vi "Chamber controller Nov 21 2016.vi"() -> ()   [LabVIEW 2014]
uses:
  <vilib>/Instr/_visa.llb/VISA Configure Serial Port (Instr).vi
  Environmental Chamber LabVIEW and Instruments/Drivers and Software/Keithley 2100 Series/Public/Configure/Configure 2 Wire Resistance.vi
  <vilib>/Utility/file.llb/Write To Spreadsheet File (string).vi
  <vilib>/Utility/file.llb/Read From Spreadsheet File (string).vi
  Environmental Chamber LabVIEW and Instruments/Drivers and Software/keithley_6430/Keithley 6430/Public/Data/Read (Single Point).vi
  Environmental Chamber LabVIEW and Instruments/Drivers and Software/LabVIEW 8.2 Drivers/keithley_24xx/Keithley 24XX/Public/Data/Read (Single Point).vi
  Environmental Chamber LabVIEW and Instruments/Drivers and Software/keithley_24xx/Keithley 24XX/Keithley 24XX.lvlib
  Environmental Chamber LabVIEW and Instruments/Drivers and Software/keithley_6430/Keithley 6430/Keithley 6430.lvlib
  Environmental Chamber LabVIEW and Instruments/Drivers and Software/Keithley 2100 Series/Keithley 2100 Series.lvlib
panel:
  in  "Arduino COMs":T1={"Arduino 1"="COM23", "Arduino 2"="COM24", "Arduino 3"="COM25", "Arduino 4"="COM26", "Arduino 5"="COM27", "Arduino 6"="COM28"}
  out "saving data?":bool
  out "ArduinoQCM\ncluster":T2 caption="Arduino QCM" {"6" format="%#_10g"; "5" format="%#_10g"; "4" format="%#_10g"; "3" format="%#_10g"; "2" format="%#_10g"; "1" format="%#_10g"}
  in  "Data logging settings":T3={"Save during sequence only"=TRUE, "Save now"=FALSE, "sec between data points"=0.0, "Current data file path"=path "", "Save sample names"={"QCM1"="", "QCM2"="", "QCM3"="", "QCM4"="", "QCM5"="", "QCM6"="", "SRS"="", "K-2420"="", "K-6430"="", "K-2100"=""}, "Experiment Notes"=""} {"sec between data points" min=0.0 max=30.0 format="%#_13g"}
  in  "Sequence cluster":T4={"Save sequence"=FALSE, "Clear sequence"=FALSE, "Import sequence file"=FALSE, "Tare elapsed time"=TRUE, "Run Sequence"=FALSE, "Stop program when sequence ends"=TRUE, "User-defined\nsequence"=[], "Sequence end time"="", "Sequence\npreview"=[], "Current\nstep"=0, "Jump to next step"=FALSE} caption="Sequence settings"
  in  "Pressure parameters cluster":T5={"valve % open"=100.0, "Desired pressure"=0.0, "Vapor sccm"=0.0, "Gas sccm"=0.0, "Valve mode"=enum."% Open", "Pressure Mode"=enum."Abs. pressure", "analyte partial pressure"=23.8, "Turbo pump\nauto on"=TRUE, "Valve position (%)"=0.0, "read pressure"=0.0, "read vapor flow"=0.0, "read gas flow"=0.0, "pressure chart"={"pressure"=0.0}} caption="Pressure settings" {"read gas flow" format="%#_3g"; "read vapor flow" format="%#_3g"; "read pressure" format="%#_7f"; "Valve position (%)" format="%#_3g"; "analyte partial pressure" min=0.0 max=100.0 step=5.0; "Gas sccm" min=0 max=200 step=5; "Vapor sccm" min=0 max=200 step=5; "Desired pressure" min=0.0 max=760.0 step=5.0; "valve % open" min=0.0 max=100.0 step=5.0 format="%#_2f"}
  out "J-KEM temp chart":dbl(graph)
  out "Elapsed time (min)":dbl
  out "State date/time":string caption="Start time"
  out "K-2100 (Ohm)":cluster{"Measurement":dbl}(graph) caption="K-2100 Ohm"
  out "K-6430":cluster{"Measurement":dbl}(graph)
  out "K-2420":cluster{"Resistance":sgl}(graph)
  in  "Gate time (sec)":enum16{"0.1", "1.0 ", "10"}(ring)=enum."1.0 "
  out "MHz":dbl format="%.7f"
  out "QCM plot":T6(graph)
  in  "Stop":bool
  in  "Clear all charts":bool
  out "O2 sensor output":dbl[](array[numeric]) caption="atm\nTorr"
  in  "rapidox O2 Sensor":bool
  in  "setnag O2 Pump":bool
  in  "Baud Rate 2":i32(ring)=2 items=["2400", "4800", "9600", "19200", "38400", "57600", "115200"]
  in  "Com Port":i32(ring) items=["Com 1", "Com 2", "Com 3", "Com 4", "Com 5", "Com 6", "COM 7", "COM 8", "COM 9", "COM 10", "COM 11", "COM 12", "com 13", "COM 14"]
  in  "Com Port 2":i32(ring) items=["Com 1", "Com 2", "Com 3", "Com 4", "Com 5", "Com 6", "COM 7", "COM 8", "COM 9", "COM 10", "COM 11", "COM 12", "com 13", "COM 14"]
  out "Waveform Chart":cluster{dbl}(graph)
  out "O2 Concentration (PPM)":dbl
  out "Waveform Chart 6":cluster{dbl}(graph)
  # "Currently Unused"
  # "100%"
  # "SRS"
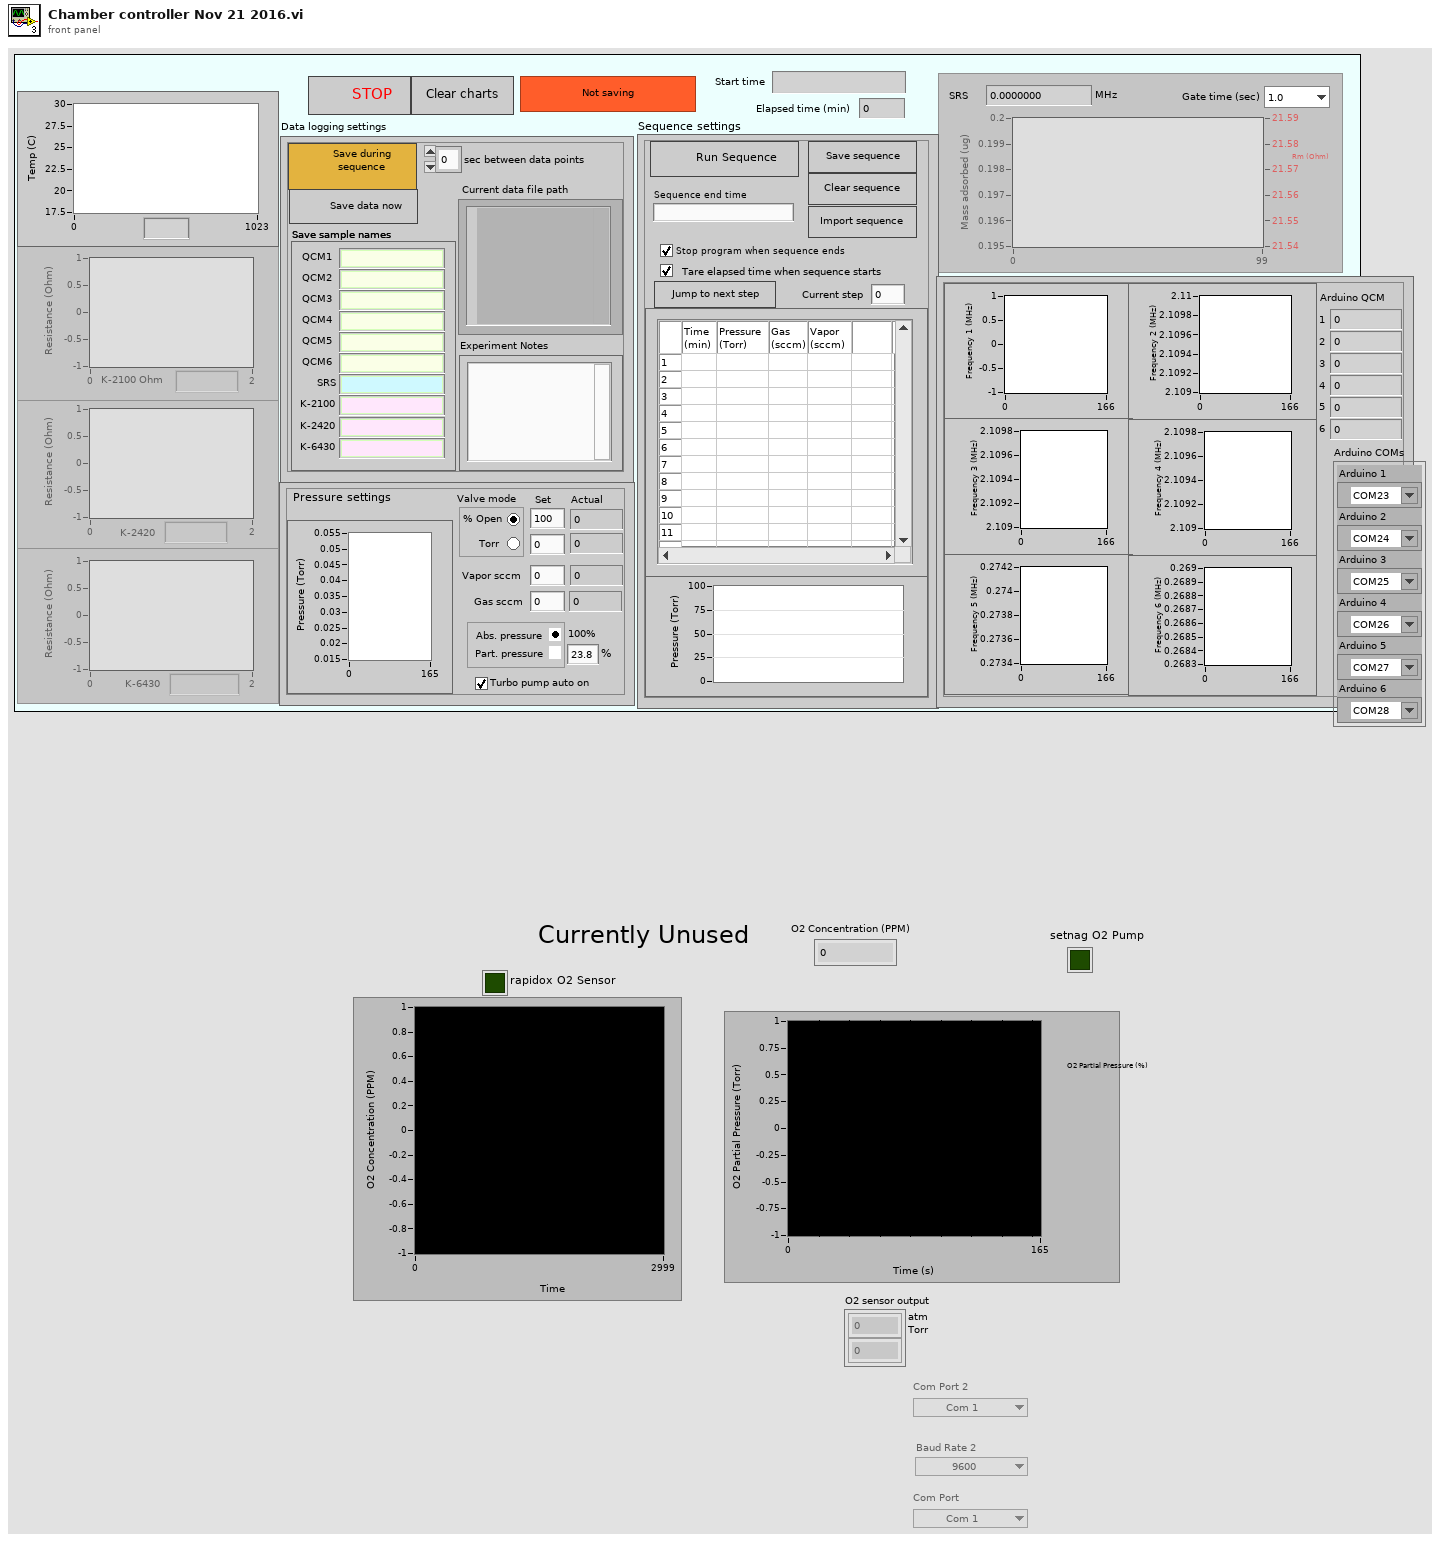
[diagram p1: front panel]
types:
  T1 = cluster{"Arduino 1":refnum<visa-resource-name>, "Arduino 2":refnum<visa-resource-name>, "Arduino 3":refnum<visa-resource-name>, "Arduino 4":refnum<visa-resource-name>, "Arduino 5":refnum<visa-resource-name>, "Arduino 6":refnum<visa-resource-name>}
  T2 = cluster{"arduino qcm 1":dbl, "1":dbl, "arduino qcm 2":dbl, "2":dbl, "arduino qcm 3":dbl, "3":dbl, "arduino qcm 4":dbl, "4":dbl, "arduino qcm 5":dbl, "5":dbl, "arduino qcm 6":dbl, "6":dbl}
  T3 = cluster{"Save during sequence only":bool, "Save now":bool, "sec between data points":dbl, "Current data file path":path, "Save sample names":cluster{"QCM1":string, "QCM2":string, "QCM3":string, "QCM4":string, "QCM5":string, "QCM6":string, "SRS":string, "K-2420":string, "K-6430":string, "K-2100":string}, "Experiment Notes":string}
  T4 = cluster{"Save sequence":bool, "Clear sequence":bool, "Import sequence file":bool, "Tare elapsed time":bool, "Run Sequence":bool, "Stop program when sequence ends":bool, "User-defined\nsequence":string[][], "Sequence end time":string, "Sequence\npreview":cluster{dbl[], dbl[]}[], "Current\nstep":i32, "Jump to next step":bool}
  T5 = cluster{"valve % open":dbl, "Desired pressure":dbl, "Vapor sccm":sgl, "Gas sccm":sgl, "Valve mode":enum32{"% Open", "Torr "}, "Pressure Mode":enum32{"Abs. pressure", " Part. pressure"}, "analyte partial pressure":dbl, "Turbo pump\nauto on":bool, "Valve position (%)":dbl, "read pressure":dbl, "read vapor flow":dbl, "read gas flow":dbl, "pressure chart":cluster{"pressure":dbl}}
  T6 = cluster{"Numeric Control":dbl, "Resistance out":dbl}
  T7 = cluster{"Keithley 6430":bool, "J-KEM":bool, "Keithley 2420":bool, "Keithley 2100":bool, "SRS QCM":bool, "Pressure control":bool, "Arduino":bool}
  T8 = enum8{"Enabled", "Disabled", "Disabled and Grayed Out"}
  T9 = enum16{"open", "open or create", "create or replace", "create", "open (read only)"}
  T10 = enum16{"no parity", "odd parity", "even parity", "mark parity", "space parity"}
  T11 = cluster{"f":dbl, "f":dbl, "f":dbl, "f":dbl, "f":dbl, "f 2":dbl}
  T12 = cluster{"String":string, "String":string, "String":string}
  T13 = cluster{"task out":refnum<k21>, "error out":errorcluster, "task out":refnum<k21>, "error out":errorcluster, "task out":refnum<k21>, "error out":errorcluster, "VISA resource name":refnum<visa-resource-name>, "error out":errorcluster}
  T14 = cluster{"task out":refnum<k21>, "error out":errorcluster, "task out":refnum<k21>, "error out":errorcluster, "task out":refnum<k21>, "error out":errorcluster, "VISA resource name out":refnum<visa-resource-name>, "error out":errorcluster}
  T15 = cluster{bool, "VISA resource name":refnum<visa-resource-name>, "error out":errorcluster}
  T16 = cluster{bool, "VISA resource name out":refnum<visa-resource-name>, "error out":errorcluster}
  T17 = cluster{"VISA resource name out":refnum<visa-resource-name>, "error out":errorcluster, "VISA resource name out":refnum<visa-resource-name>, "error out":errorcluster, "VISA resource name out":refnum<visa-resource-name>, "error out":errorcluster, "VISA resource name out":refnum<visa-resource-name>, "error out":errorcluster, "VISA resource name out":refnum<visa-resource-name>, "error out":errorcluster, "VISA resource name out 2":refnum<visa-resource-name>, "error out 2":errorcluster}
  T18 = cluster{bool, cluster{"task out":refnum<k21>, "error out":errorcluster, "task out":refnum<k21>, "error out":errorcluster, "task out":refnum<k21>, "error out":errorcluster, "VISA resource name out":refnum<visa-resource-name>, "error out":errorcluster}}
  T19 = cluster{"Boolean":bool, "VISA resource name out":refnum<visa-resource-name>, "error out":errorcluster}
  T20 = cluster{bool, "VISA out":refnum<visa-resource-name>, "error out":errorcluster}
  T21 = cluster{"Boolean":bool, "VISA out":refnum<visa-resource-name>, "error out":errorcluster}
  T22 = cluster{"Numeric Control":dbl, "Cluster":cluster{"Numeric Control":dbl}, "String":string, "error out":errorcluster}
  T23 = cluster{bool, "Com Port":i32, "Numeric Control out":dbl}
  T24 = cluster{"Arduino address":refnum<visa-resource-name>, "error in (no error)":errorcluster, "Arduino address 2":refnum<visa-resource-name>, "error in (no error) 2":errorcluster, "Arduino address 3":refnum<visa-resource-name>, "error in (no error) 3":errorcluster, "Arduino address 4":refnum<visa-resource-name>, "error in (no error) 4":errorcluster, "Arduino address 5":refnum<visa-resource-name>, "error in (no error) 5":errorcluster, "Arduino address 6":refnum<visa-resource-name>, "error in (no error) 6":errorcluster}
  T25 = cluster{"mean":string, "mean":string, "mean":string, "mean":string, "mean":string, "mean":string}
  T26 = cluster{"String data out":string, string, string, string}
  T27 = cluster{"valve % open":dbl, "Desired pressure":dbl, "Vapor sccm":sgl, "Gas sccm":sgl, "Valve mode":enum32{"% Open", "Torr "}, "Pressure Mode":enum32{"Abs. pressure", " Part. pressure"}, "analyte partial pressure":dbl, "Turbo pump\nauto on":bool}
  T28 = cluster{"User-defined\nsequence":string[][], "Present (s)":dbl, "current  step # in":i32, "sequence end time in":timestamp}
  T29 = cluster{"current  step # in":i32, "sequence end time in":timestamp, "Boolean":bool}
  T30 = cluster{"press/RH/gas/vapor":cluster{"pressure":string, "RH":string, "gas flow":string, "vapor flow":string}, "Cluster":cluster{"Valve position (%)":dbl, "read pressure":dbl, "read vapor flow":dbl, "read gas flow":dbl}}
  T31 = cluster{"Boolean":bool, "DAQ IDs in":cluster{"task out":refnum<k21>, "error out":errorcluster, "task out":refnum<k21>, "error out":errorcluster, "task out":refnum<k21>, "error out":errorcluster, "VISA Refnum out":refnum<visa-resource-name>, "error out":errorcluster}}
  T32 = cluster{"mean":dbl, "mean":dbl, "mean":dbl, "mean":dbl, "mean":dbl, "mean":dbl}
  T33 = cluster{"f":dbl, "f":dbl, "f":dbl, "f":dbl, "f":dbl}[]
  T34 = cluster{"pressure":string, "RH":string, "gas flow":string, "vapor flow":string}
  T35 = cluster{"Valve position (%)":dbl, "read pressure":dbl, "read vapor flow":dbl, "read gas flow":dbl}
  T36 = cluster{dbl, dbl, dbl, dbl, dbl, dbl, dbl, dbl, dbl, dbl, dbl, dbl}
  T37 = cluster{"QCM1":string, "QCM2":string, "QCM3":string, "QCM4":string, "QCM5":string, "QCM6":string, "SRS":string, "K-2420":string, "K-6430":string, "K-2100":string}
  T38 = cluster{"task out":refnum<k21>, "error out":errorcluster, "task out":refnum<k21>, "error out":errorcluster, "task out":refnum<k21>, "error out":errorcluster, "VISA Refnum out":refnum<visa-resource-name>, "error out":errorcluster}
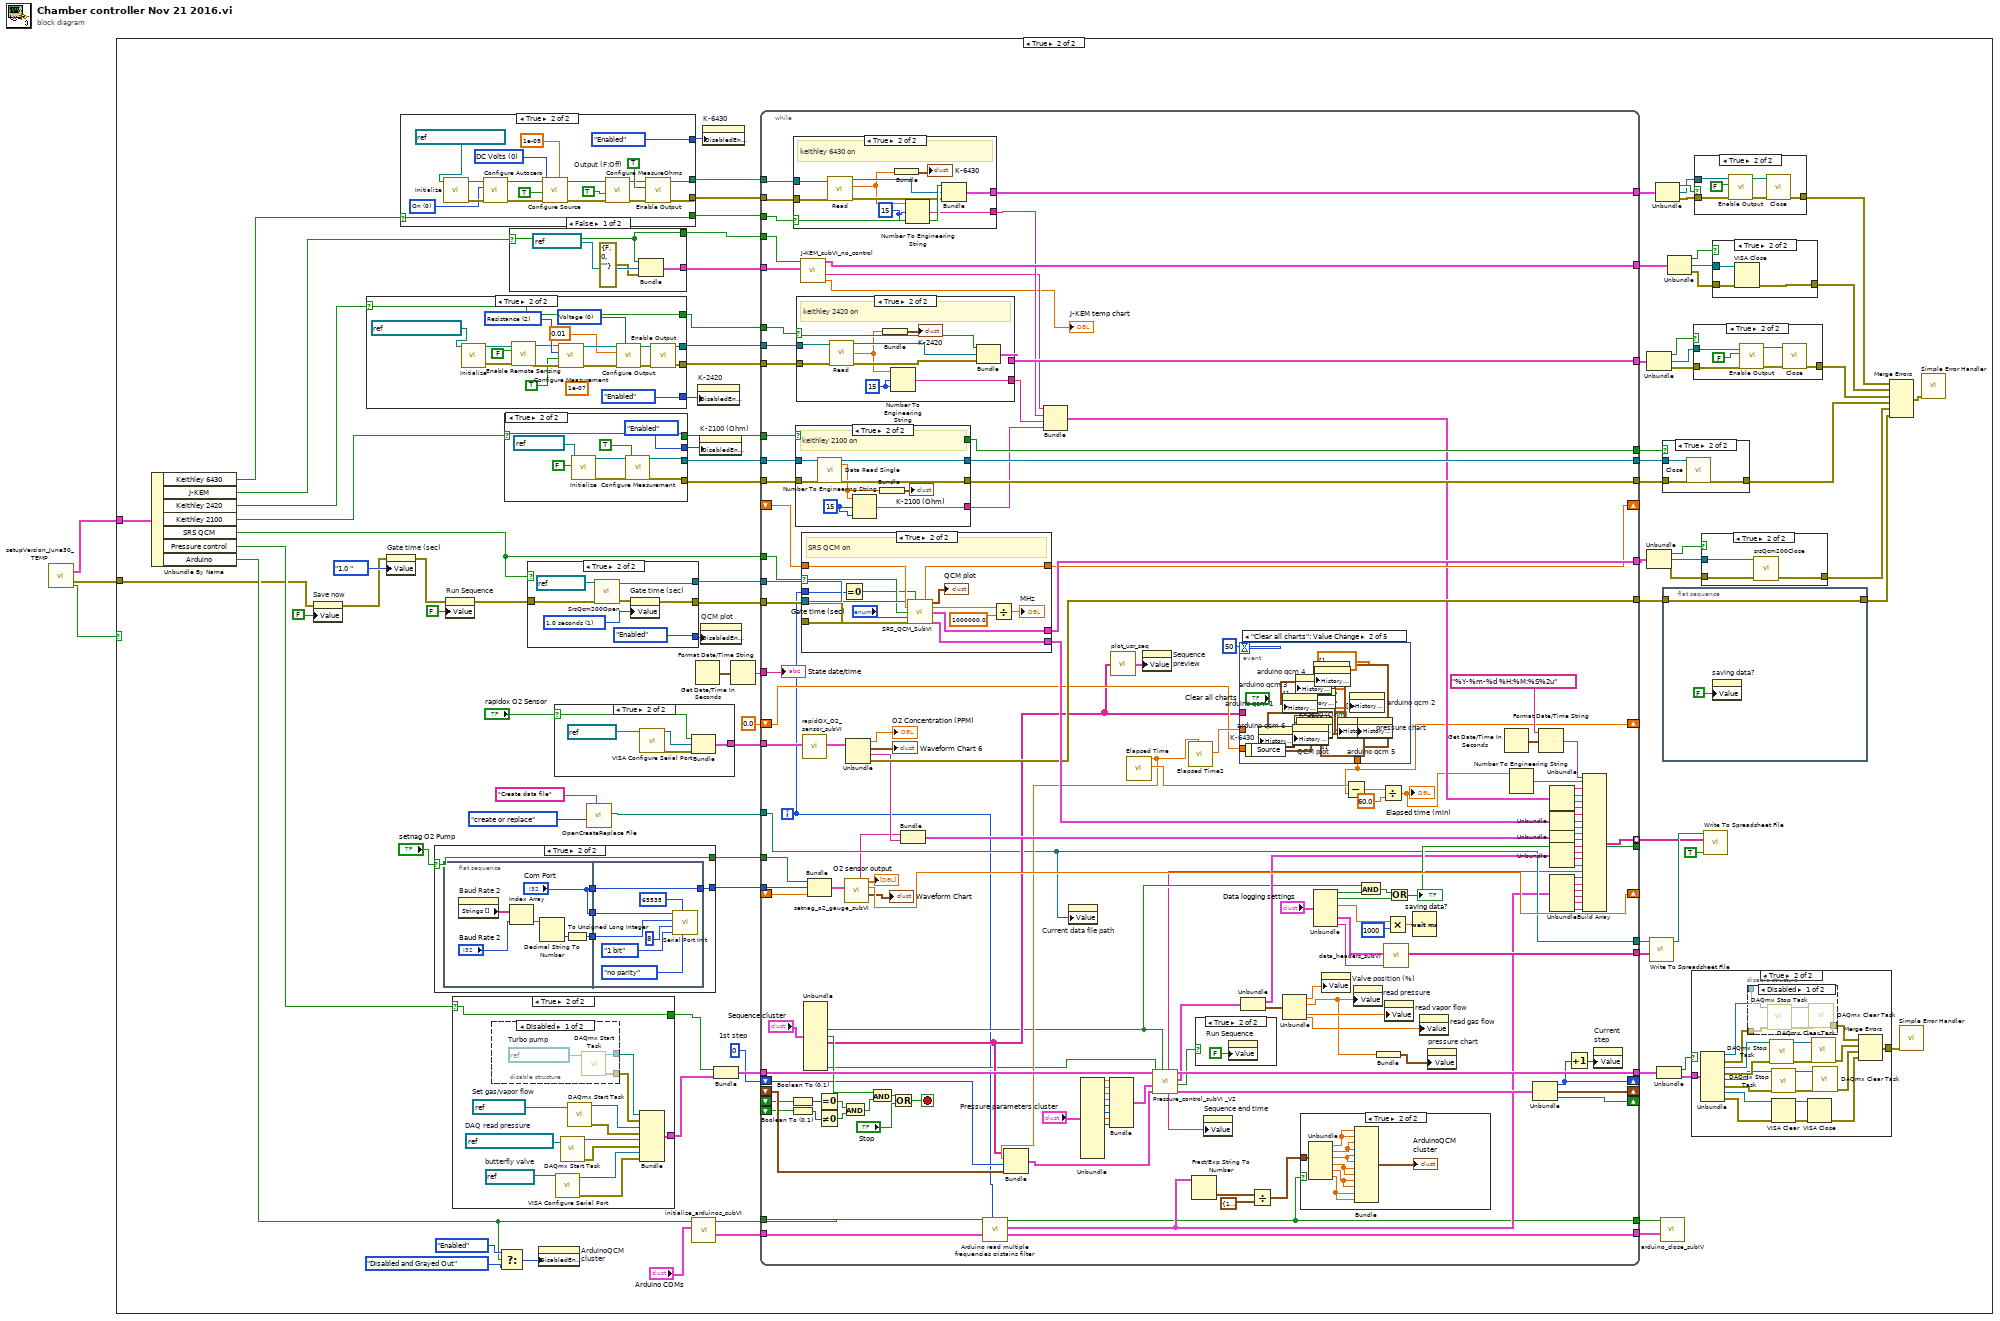
[diagram p0: block diagram]
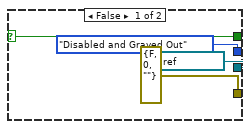
[diagram p4: hidden frame]
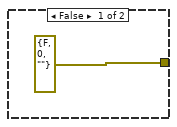
[diagram p5: hidden frame]
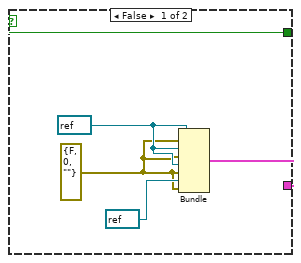
[diagram p7: hidden frame]
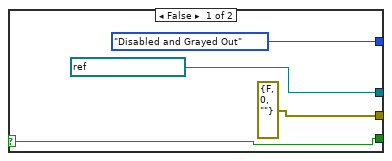
[diagram p10: hidden frame]
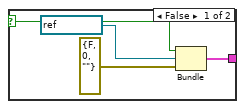
[diagram p11: hidden frame]
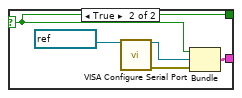
[diagram p13: hidden frame]
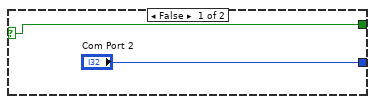
[diagram p14: hidden frame]
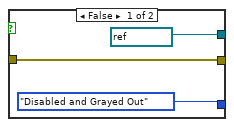
[diagram p16: hidden frame]
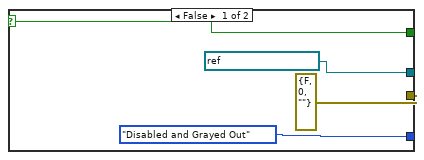
[diagram p18: hidden frame]
diagram:
  n1 = call "setupVersion_June30_TEMP.vi"() -> ("Instruments on/off"=w1:T7, "error IO"=w2:errorcluster, "OK"=w3:bool)  [unwired: 13 in]
  n2 = case shown="True" w3 {
    tunnel: w2 -> [_ w8]
    tunnel: w1 -> [_ w16]
    frame False {
    }
    frame True {
      w28 = 0  # 1st step
      n3 = Unbundle By Name(w16) -> ("Keithley 6430"=w15:bool, "J-KEM"=w14:bool, "Keithley 2420"=w13:bool, "Keithley 2100"=w12:bool, "SRS QCM"=w11:bool, "Pressure control"=w10:bool, "Arduino"=w9:bool)
      n4 = property on="Save now" class="Bool (strict)"(error in=w8, "Value"=FALSE) -> (error out=w7:errorcluster)  [unwired: 1 in, 1 out]
      n5 = case shown="True" w13 {
        selector: w13 -> [w254 w258]
        tunnel: [refnum<visa-resource-name> "GPIB1::24::INSTR" ("VISA resource name") w267] -> w92
        tunnel: [errorcluster {"status"=FALSE, "code"=0, "source"=""} ("error out") w262] -> w91
        tunnel: [T8."Disabled and Grayed Out" ("Disabled") T8."Enabled" ("Disabled")] -> w55
        tunnel: [w254 w258] -> w48
        frame False {
        }
        frame True {
          (unwired) 1e-07 ("Manual Range (1.0)")
          w269 = u16 0 items=["Voltage", "Current"] ("Source Mode  (0: Voltage)")
          w274 = u16 2 items=["Volts", "Current", "Resistance"] ("Function (0: Volts)")
          n6 = call "Initialize.vi"("VISA resource name"=refnum<visa-resource-name> "GPIB1::24::INSTR") -> ("error out"=w263:errorcluster, "VISA resource name out"=w266:refnum<visa-resource-name>)  [unwired: 9 in]
          n7 = call "Enable Remote Sensing.vi"("error in (no error)"=w263, "Enable Remote Sensing (T: Enable)"=FALSE ("4-wire?"), "VISA resource name"=w266) -> ("error out"=w264:errorcluster, "VISA resource name out"=w265:refnum<visa-resource-name>)  [unwired: 7 in]
          n8 = call "Configure Measurement.vi"("error in (no error)"=w264, "Enable Auto Range (T:Enable)"=TRUE, "Function (0: Volts)"=w274, "VISA resource name"=w265) -> ("error out"=w273:errorcluster, "VISA resource name out"=w272:refnum<visa-resource-name>)  [unwired: 6 in]
          n9 = call "Configure Output.vi"("Source Mode  (0: Voltage)"=w269, "error in (no error)"=w273, "Output Level (0)"=0.01 ("Applied Voltage (V)"), "VISA resource name"=w272) -> ("error out"=w271:errorcluster, "VISA resource name out"=w270:refnum<visa-resource-name>)  [unwired: 6 in]
          n10 = call "Enable Output.vi"("error in (no error)"=w271, "VISA resource name"=w270) -> ("error out"=w262:errorcluster, "VISA resource name out"=w267:refnum<visa-resource-name>)  [unwired: 8 in]
        }
      }
      n11 = property on="Gate time (sec)" class="Enum (strict)"(error in=w7, "Value"=enum16{"0.1", "1.0 ", "10"}."1.0 " ("Gate time (sec)")) -> (error out=w17:errorcluster)  [unwired: 1 in, 1 out]
      n12 = case shown="True" w15 {
        selector: w15 -> [w168 w172]
        tunnel: [refnum<visa-resource-name> "GPIB0::29::INSTR" ("VISA resource name") w185] -> w61
        tunnel: [errorcluster {"status"=FALSE, "code"=0, "source"=""} ("error out") w186] -> w60
        tunnel: [T8."Disabled and Grayed Out" ("Disabled") T8."Enabled" ("Disabled")] -> w54
        tunnel: [w168 w172] -> w47
        frame False {
        }
        frame True {
          w174 = u16 0 items=["DC Volts", "DC Current"] ("Source Function (0: DC Volts)")
          w181 = u16 0 items=["On", "Off", "Once"] ("Autozero  (0: On)")
          w189 = TRUE  # Output (F:Off)
          n13 = call "Initialize.vi"("VISA resource name"=refnum<visa-resource-name> "GPIB0::30::INSTR") -> ("error out"=w182:errorcluster, "VISA resource name out"=w183:refnum<visa-resource-name>)  [unwired: 4 in, 5 out]
          n14 = call "Configure Autozero.vi"("error in (no error)"=w182, "Autozero  (0: On)"=w181, "VISA resource name"=w183) -> ("error out"=w177:errorcluster, "VISA resource name out"=w179:refnum<visa-resource-name>)  [unwired: 7 in]
          n15 = call "Configure Source.vi"("I-Source Level [A]"=1e-09, "error in (no error)"=w177, "Auto Range (T:Enable)"=TRUE, "Source Function (0: DC Volts)"=w174, "VISA resource name"=w179) -> ("error out"=w176:errorcluster, "VISA resource name out"=w178:refnum<visa-resource-name>)  [unwired: 5 in]
          n16 = call "Configure MeasureOhms.vi"("error in (no error)"=w176, "Auto Range (T:Enable)"=TRUE, "VISA resource name"=w178) -> ("error out"=w190:errorcluster, "VISA resource name out"=w188:refnum<visa-resource-name>)  [unwired: 3 in, 4 out]
          n17 = call "Enable Output.vi"("error in (no error)"=w190, "Enable Output (F:Off)"=w189, "VISA resource name"=w188) -> ("error out"=w186:errorcluster, "VISA resource name out"=w185:refnum<visa-resource-name>)  [unwired: 7 out]
        }
      }
      n18 = case shown="True" "setnag O2 Pump" {
        selector: "setnag O2 Pump" -> [w213 w215]
        tunnel: ["Com Port 2" w216] -> w88
        tunnel: [w213 w215] -> w36
        frame False {
        }
        frame True {
          n19 = flat-sequence {
            tunnel: ["Com Port"] -> w219
            tunnel: [w221] -> w218
            tunnel: ["Com Port"] -> w217
            tunnel: w219 -> [w227]
            tunnel: w218 -> [w226]
            tunnel: w217 -> [w228]
            tunnel: [w228] -> w216
            frame #0 {
              n20 = property on="Baud Rate 2" class="Ring (strict)"() -> ("Strings []"=w223:string[])  [unwired: 2 in, 2 out]
              n21 = Index Array(array=w223, index="Baud Rate 2") -> (element=w224:string)
              n22 = Decimal String To Number(string=w224) -> (number=w222:i32)  [unwired: 2 in, 1 out]
              n23 = To Unsigned Long Integer(number=w222) -> (unsigned 32bit integer=w221:u32)
            }
            frame #1 {
              n24 = call <vilib>:"Serial Port Init.vi"("parity"=T10."no parity", "buffer size"=u16 65535, "stop bits"=enum16{"1 bit", "1.5 bits", "2 bits"}."1 bit", "data bits"=u16 8, "baud rate"=w226, "port number"=w227) -> ()  [unwired: 1 in, 1 out]
            }
          }
        }
      }
      n25 = property on="Run Sequence" class="Bool (strict)"(error in=w17, "Value"=FALSE) -> (error out=w23:errorcluster)  [unwired: 1 in, 1 out]
      n26 = case shown="True" w10 {
        selector: w10 -> [w140 w145]
        tunnel: [w141 w147] -> w30
        tunnel: [w140 w145] -> w31
        frame False {
          w143 = refnum<k21> refnum ("task out")
          w142 = errorcluster {"status"=FALSE, "code"=0, "source"=""} ("error out")
          n27 = Bundle("task out"=w143, "error out"=w142, "task out"=w143, "error out"=w142, "task out"=w143, "error out"=w142, "VISA resource name"=refnum<visa-resource-name> refnum, "error out"=w142) -> (w141:T13)  [unwired: 1 in]
        }
        frame True {
          w155 = refnum<visa-resource-name> "COM5"  # butterfly valve
          w156 = refnum<k21> "Setflow"  # Set gas/vapor flow
          w157 = refnum<k21> "AllDaqReadings"  # DAQ read pressure
          n28 = disable-structure shown="Disabled" {
            disable-tunnel: [w159 _] -> w154
            disable-tunnel: [w158 _] -> w153
            frame Disabled {
              w160 = refnum<k21> "TurboON"  # Turbo pump
              n29 = call <vilib>:"DAQmx Start Task.vi"("task/channels in"=w160) -> ("task out"=w159:refnum<k21>, "error out"=w158:errorcluster)  [unwired: 13 in]
            }
            frame Enabled {
            }
          }
          n30 = call-poly "VISA Configure Serial Port"("VISA resource name"=w155) -> ("VISA resource name out"=w148:refnum<visa-resource-name>, "error out"=w146:errorcluster)  [unwired: 13 in]
          n31 = call <vilib>:"DAQmx Start Task.vi"("task/channels in"=w157) -> ("task out"=w150:refnum<k21>, "error out"=w149:errorcluster)  [unwired: 13 in]
          n32 = call <vilib>:"DAQmx Start Task.vi"("task/channels in"=w156) -> ("task out"=w152:refnum<k21>, "error out"=w151:errorcluster)  [unwired: 13 in]
          n33 = Bundle("task out"=w154, "error out"=w153, "task out"=w152, "error out"=w151, "task out"=w150, "error out"=w149, "VISA resource name out"=w148, "error out"=w146) -> (w147:T14)  [unwired: 1 in]
        }
      }
      n34 = Select(t=T8."Enabled" ("Disabled"), s=w9, f=T8."Disabled and Grayed Out" ("Disabled")) -> (s? t:f=w22:T8)
      n35 = case shown="True" w12 {
        selector: w12 -> [w102 w107]
        tunnel: [refnum<visa-resource-name> "K-2100" ("VISA resource name out") w110] -> w45
        tunnel: [errorcluster {"status"=FALSE, "code"=0, "source"=""} ("error out") w109] -> w44
        tunnel: [w102 w107] -> w43
        tunnel: [T8."Disabled and Grayed Out" ("Disabled") T8."Enabled" ("Disabled")] -> w38
        frame False {
        }
        frame True {
          n36 = call "Initialize.vi"("VISA resource name"=refnum<visa-resource-name> "K-2100", "Reset? (T: Reset)"=FALSE) -> ("VISA resource name out"=w111:refnum<visa-resource-name>, "error out"=w108:errorcluster)  [unwired: 16 in]
          n37 = call-poly "Configure Measurement.vi"("VISA resource name"=w111, "error in (no error)"=w108, "Auto Range? (T: Auto)"=TRUE) -> ("VISA resource name out"=w110:refnum<visa-resource-name>, "error out"=w109:errorcluster)  [unwired: 15 in]
        }
      }
      n38 = case shown="False" w14 {
        selector: w14 -> [w204 w209]
        tunnel: [w205 w210] -> w77
        tunnel: [w204 w209] -> w71
        frame False {
          n39 = Bundle(w204, "VISA resource name"=refnum<visa-resource-name> "COM3", "error out"=errorcluster {"status"=FALSE, "code"=0, "source"=""}) -> (w205:T15)  [unwired: 1 in]
        }
        frame True {
          n40 = call-poly "VISA Configure Serial Port"("VISA resource name"=refnum<visa-resource-name> "COM3") -> ("VISA resource name out"=w211:refnum<visa-resource-name>, "error out"=w208:errorcluster)  [unwired: 13 in]
          n41 = Bundle(w209, "VISA resource name out"=w211, "error out"=w208) -> (w210:T16)  [unwired: 1 in]
        }
      }
      n42 = case shown="True" w11 {
        tunnel: [refnum<visa-resource-name> "COM6" ("VISA in") w243] -> w90
        tunnel: [w238 w240] -> w89
        tunnel: w23 -> [w238 w245]
        tunnel: [T8."Disabled and Grayed Out" ("Disabled") T8."Enabled" ("Disabled")] -> w56
        frame False {
        }
        frame True {
          w242 = u16 1 items=["0.1 seconds", "1.0 seconds", "10.0 seconds"] ("Gate time")
          n43 = call "SrsQcm200Open.vi"("error in"=w245, "VISA in"=refnum<visa-resource-name> "COM6") -> ("error out"=w241:errorcluster, "VISA out"=w243:refnum<visa-resource-name>)  [unwired: 3 in]
          n44 = property on="Gate time (sec)" class="Enum (strict)"(error in=w241, "Value"=w242) -> (error out=w240:errorcluster)  [unwired: 1 in, 1 out]
        }
      }
      n45 = property on="ArduinoQCM\ncluster" class="Clust (strict)"("DisabledEnum"=w22) -> ()  [unwired: 2 in, 2 out]
      n46 = case shown="True" "rapidox O2 Sensor" {
        selector: "rapidox O2 Sensor" -> [w191 w196]
        tunnel: [w192 w197] -> w67
        frame False {
          n47 = Bundle(w191, "VISA resource name"=refnum<visa-resource-name> "COM7", "error out"=errorcluster {"status"=FALSE, "code"=0, "source"=""}) -> (w192:T15)  [unwired: 1 in]
        }
        frame True {
          n48 = call-poly "VISA Configure Serial Port"("VISA resource name"=refnum<visa-resource-name> "COM7") -> ("VISA resource name out"=w198:refnum<visa-resource-name>, "error out"=w195:errorcluster)  [unwired: 13 in]
          n49 = Bundle(w196, "VISA resource name out"=w198, "error out"=w195) -> (w197:T16)  [unwired: 1 in]
        }
      }
      n50 = call "OpenCreateReplace File.vi"("prompt"="Create data file", "function (open:0)"=T9."create or replace") -> ("new file path"=w46:path)  [unwired: 6 in, 3 out]
      n51 = call "initialize_arduinos_subVI.vi"("arduino 1-6 addresses"="Arduino COMs", "arduinos on?"=w9) -> ("arduino addresses/errors"=w32:T17, "arduinos on/off"=w52:bool)  [unwired: 8 in]
      n52 = Get Date/Time In Seconds() -> (seconds since 1Jan1904=w94:timestamp)
      n53 = property on="K-2420" class="WFChart (strict)"("DisabledEnum"=w55) -> ()  [unwired: 2 in, 2 out]
      n54 = property on="K-2100 (Ohm)" class="WFChart (strict)"("DisabledEnum"=w38) -> ()  [unwired: 2 in, 2 out]
      n55 = property on="QCM plot" class="WFChart (strict)"("DisabledEnum"=w56) -> ()  [unwired: 2 in, 2 out]
      n56 = property on="K-6430" class="WFChart (strict)"("DisabledEnum"=w54) -> ()  [unwired: 2 in, 2 out]
      n57 = Bundle(w31, w30) -> (w29:T18)  [unwired: 1 in]
      n58 = Format Date/Time String(seconds (now)=w94) -> (date/time string=w35:string)  [unwired: 2 in]
      n59 = while {
        shift-right: [w421] -> _
        shift-left: _ -> [w349]
        tunnel: [w405] -> w53 mode=indexing if=w372
        tunnel: w48 -> [w410]
        tunnel: w92 -> [w420]
        tunnel: w91 -> [w419]
        tunnel: w90 -> [w418]
        tunnel: w89 -> [w417]
        tunnel: w11 -> [w416]
        tunnel: w36 -> [w351]
        tunnel: w88 -> [w352]
        tunnel: [w415] -> w85
        tunnel: [w414] -> w81
        tunnel: w77 -> [w413]
        tunnel: [w412] -> w76
        tunnel: w71 -> [w411]
        tunnel: w67 -> [w360]
        tunnel: [w356] -> w5
        tunnel: [w291] -> w66
        tunnel: w46 -> [w291]
        shift-right: [w403] -> _
        shift-left: _ -> [w404]
        tunnel: w61 -> [w409]
        tunnel: w60 -> [w408]
        tunnel: [w407] -> w59
        tunnel: [w372] -> _
        tunnel: w52 -> [w278]
        tunnel: w32 -> [w281]
        tunnel: [w277] -> w50
        tunnel: [w279] -> w51
        tunnel: [w391] -> w49
        tunnel: w47 -> [w384]
        tunnel: w45 -> [w371]
        tunnel: w44 -> [w370]
        tunnel: w43 -> [w369]
        tunnel: [w368] -> w42
        tunnel: [w367] -> w41
        tunnel: [w366] -> w40
        shift-right: [w343] -> _
        shift-left: 0.0 ("Elapsed Time (s)") -> [w344]
        tunnel: w35 -> [w334]
        tunnel: w29 -> [w316]
        shift-right: [w286] -> _
        shift-left: w28 -> [w305]
        shift-right: [w311] -> _
        shift-left: _ -> [w309]
        shift-right: [w310] -> _
        shift-left: _ -> [w308]
        shift-left: _ -> [w307]
        tunnel: [w303] -> w27
        i -> [w276]
        stop <- w374 stop-if-true
        n60 = Boolean To (0,1)(Boolean=w308) -> (0, 1=w382:i16)
        n61 = Boolean To (0,1)(Boolean=w307) -> (0, 1=w381:i16)
        n62 = case "Keithley 6430" shown="True" w384 {
          selector: w384 -> [w456 w467]
          tunnel: w409 -> [w455 w464]
          tunnel: w408 -> [w454 w463]
          tunnel: ["" w466] -> w355
          tunnel: [w453 w465] -> w407
          frame False {
            # "keithley 6430 off"
            n63 = Bundle(w456, "VISA resource name out"=w455, "error out"=w454) -> (w453:T16)  [unwired: 1 in]
          }
          frame True {
            w458 = i16 15 ("width (-)")
            # "keithley 6430 on"
            n64 = call-poly "Read.vi"("error in (no error)"=w463, "VISA resource name"=w464) -> ("error out"=w462:errorcluster, "Measurement"=w460:dbl, "VISA resource name out"=w461:refnum<visa-resource-name>)  [unwired: 1 in, 6 out]
            n65 = Bundle("Measurement"=w460) -> (→"K-6430":cluster{"Measurement":dbl})  [unwired: 1 in]
            n66 = Number To Engineering String(2:w458, 3:w458, 4:w460) -> (0:w466:string)  [unwired: 1 in]
            n67 = Bundle(w467, "VISA resource name out"=w461, "error out"=w462) -> (w465:T16)  [unwired: 1 in]
          }
        }
        n68 = case shown="True" w369 {
          selector: w369 -> [w432 w437]
          tunnel: [w433 w444] -> w367
          tunnel: [w434 w443] -> w366
          tunnel: w371 -> [w433 w442]
          tunnel: w370 -> [w434 w441]
          tunnel: ["" w439] -> w353
          tunnel: [w432 w437] -> w368
          frame False {
            # "keithley 2100 off"
          }
          frame True {
            w436 = i16 15 ("width (-)")
            # "keithley 2100 on"
            n69 = call "Data Read Single.vi"("VISA resource name"=w442, "error in (no error)"=w441) -> ("VISA resource name out"=w444:refnum<visa-resource-name>, "Measurement"=w440:dbl, "error out"=w443:errorcluster)  [unwired: 15 in]
            n70 = Number To Engineering String ("elapsed time (min)")(2:w436, 3:w436, 4:w440) -> (0:w439:string)  [unwired: 1 in]
            n71 = Bundle("Measurement"=w440) -> (→"K-2100 (Ohm)":cluster{"Measurement":dbl})  [unwired: 1 in]
          }
        }
        n72 = case "Keithley 2420" shown="True" w410 {
          selector: w410 -> [w471 w480]
          tunnel: w420 -> [w470 w475]
          tunnel: w419 -> [w469 w474]
          tunnel: [w468 w478] -> w415
          tunnel: ["" w477] -> w354
          frame False {
            # "keithley 2420 off"
            n73 = Bundle(w471, "VISA resource name out"=w470, "error out"=w469) -> (w468:T16)  [unwired: 1 in]
          }
          frame True {
            w473 = i16 15 ("width (-)")
            # "keithley 2420 on"
            n74 = call-poly "Read.vi"("VISA resource name"=w475, "error in (no error)"=w474) -> ("VISA resource name out"=w481:refnum<visa-resource-name>, "Resistance"=w476:sgl, "error out"=w479:errorcluster)  [unwired: 7 in, 4 out]
            n75 = Bundle("Resistance"=w476) -> (→"K-2420":cluster{"Resistance":sgl})  [unwired: 1 in]
            n76 = Number To Engineering String(2:w473, 3:w473, 4:w476) -> (0:w477:string)  [unwired: 1 in]
            n77 = Bundle(w480, "VISA resource name out"=w481, "error out"=w479) -> (w478:T16)  [unwired: 1 in]
          }
        }
        n78 = call "J-KEM_subVI_no_control.vi"("Address in"=w413, "J-KEM on?"=w411) -> ("Temp (C)"=→"J-KEM temp chart":dbl, "String data out"=w342:string, "Address out"=w412:T19)  [unwired: 6 in, 1 out]
        n79 = case "SRS QCM" shown="True" w416 {
          selector: w416 -> [w485 w496]
          tunnel: w418 -> [w488 w498]
          tunnel: w417 -> [w487 w499]
          tunnel: [w486 w502] -> w414
          tunnel: w404 -> [w483 w501]
          tunnel: [w483 w500] -> w403
          tunnel: [T12 {"String"="", "String"="", "String"=""} ("M,F,MR output cluster") w495] -> w396
          tunnel: w276 -> [_ w489]
          frame False {
            # "SRS QCM off"
            n80 = Bundle(w485, "VISA out"=w488, "error out"=w487) -> (w486:T20)  [unwired: 1 in]
          }
          frame True {
            # "SRS QCM on"
            n81 = Equal To 0?(x=w489) -> (x = 0?=w490:bool)
            n82 = call "SRS_QCM_SubVI.vi"("VISA Refnum in"=w498, "first iteration?"=w490, "Frequency out 3"=w501, "Boolean 2"=w496, "Gate time"="Gate time (sec)", "error in (no error)"=w499) -> ("Frequency out 2"=w500:dbl, "Cluster"=→"QCM plot":T6, "Frequency out"=w491:dbl, "Cluster 2"=w502:T21, "M,F,MR output cluster"=w495:T12)  [unwired: 2 in, 3 out]
            n83 = Divide(x=w491, y=1000000.0) -> (x/y=→"MHz":dbl)
          }
        }
        n84 = call "rapidOX_O2_sensor_subVI.vi"("rapid ox info in"=w360) -> ("rapidox info out"=w359:T22)  [unwired: 10 in]
        n85 = Unbundle("Sequence cluster") -> ("Run Sequence"=w297:bool, "Stop program when sequence ends"=w306:bool, "User-defined\nsequence"=w301:string[][], "Jump to next step"=w287:bool)  [unwired: 7 out]
        n86 = Bundle(w351, "Com Port"=w352, "Numeric Control out"=w349) -> (w350:T23)  [unwired: 1 in]
        n87 = Equal To 0?(x=w382) -> (x = 0?=w379:bool)
        n88 = Not Equal To 0?(x=w381) -> (x != 0?=w380:bool)
        n89 = And(x=w379, y=w380) -> (x .and. y?=w373:bool)
        n90 = call "setnag_o2_gauge_subVI.vi"("setnag info in"=w350) -> ("Cluster"=→"Waveform Chart":cluster{"Numeric Control":dbl}, "Numeric Control out"=w421:dbl, "Array"=→"O2 sensor output":dbl[], "String"=w288:string)  [unwired: 7 in]
        n91 = Unbundle(w359) -> ("Numeric Control"=→"O2 Concentration (PPM)":dbl, "Cluster"=→"Waveform Chart 6":cluster{"Numeric Control":dbl}, "String"=w333:string, "error out"=w356:errorcluster)
        n92 = And(x=w306, y=w373) -> (x .and. y?=w347:bool)
        n93 = Or(x=w347, y="Stop") -> (x .or. y?=w374:bool)
        n94 = Bundle("String"=w288, "String"=w333) -> (w332:cluster{"String":string, "String":string})  [unwired: 1 in]
        n95 = call "Arduino read multiple frequencies cristains filter.vi"("main loop iteration number"=w276, "arduino addresses in"=w281, "arduinos on?"=w278) -> ("arduino addresses out"=w279:T24, "arduino frequencies out"=w280:T25, "arduinos on"=w277:bool)  [unwired: 6 in]
        n96 = Bundle("String data out"=w342, w355, w354, w353) -> (w348:T26)  [unwired: 1 in]
        n97 = property on="Current data file path" class="Path"("Value"=w291) -> ()  [unwired: 2 in, 2 out]
        n98 = Unbundle("Pressure parameters cluster") -> ("valve % open"=w321:dbl, "Desired pressure"=w323:dbl, "Vapor sccm"=w324:sgl, "Gas sccm"=w325:sgl, "Valve mode"=w326:enum32{"% Open", "Torr "}, "Pressure Mode"=w327:enum32{"Abs. pressure", " Part. pressure"}, "analyte partial pressure"=w328:dbl, "Turbo pump\nauto on"=w329:bool)  [unwired: 5 out]
        n99 = Bundle("valve % open"=w321, "Desired pressure"=w323, "Vapor sccm"=w324, "Gas sccm"=w325, "Valve mode"=w326, "Pressure Mode"=w327, "analyte partial pressure"=w328, "Turbo pump\nauto on"=w329) -> (w320:T27)  [unwired: 1 in]
        n100 = call "plot_usr_seq.vi"("User-defined sequence"=w301) -> ("Sequence Preview"=w293:cluster{dbl[], dbl[]}[])
        n101 = call "Elapsed Time"() -> ("Present (s)"=w313:dbl, "Elapsed Time (s)"=w362:dbl)  [unwired: 12 in, 6 out]
        n102 = Bundle("User-defined\nsequence"=w301, "Present (s)"=w313, "current  step # in"=w305, "sequence end time in"=w309) -> (w314:T28)  [unwired: 1 in]
        n103 = property on="Sequence\npreview" class="XYGraph (strict)"("Value"=w293) -> ()  [unwired: 2 in, 2 out]
        n104 = call "Pressure_control_subVI _V2.vi"("Run Sequence"=w297, "user sequence, present (s) in, current step in, seq time in"=w314, "pressure parameters in"=w320, "Jump to next step"=w287, "pressure control on? / DAQ IDs/errors in"=w316) -> ("current step # out, shift register time out, seq button on?"=w312:T29, "sequence over? USE THIS TO REINITIALIZE RUN SEQUENCE BUTTON SO PROGRAM ENDS"=w302:bool, "save press/RH/gasflow/vaporflow - read valve position/pressure/vaporflow/gasflow"=w300:T30, "pressure control on out, DAQ IDs/errors out"=w303:T31, "sequence end date/time string"=w304:string, "pressure_setpoint"=w283:string)  [unwired: 1 in]
        n105 = call "Elapsed Time2"("Set Start Time (s)"=w313) -> ("Elapsed Time (s)"=w345:dbl)  [unwired: 11 in, 7 out]
        n106 = Fract/Exp String To Number(string=w280) -> (number=w390:T32)  [unwired: 3 in, 1 out]
        n107 = case shown="True" w302 {
          frame False {
          }
          frame True {
            n108 = property on="Run Sequence" class="Bool (strict)"("Value"=FALSE ("Run Sequence")) -> ()  [unwired: 2 in, 2 out]
          }
        }
        n109 = property on="Sequence end time" class="Str"("Value"=w304) -> ()  [unwired: 2 in, 2 out]
        n110 = event shown="[1] \"Clear all charts\": Value Change" {
          selector: _ -> [_ _ _ _ _]
          dyn-events: _ -> [_ _ _ _ _]
          timeout: 50 -> [_ _ _ _ _]
          tunnel: w301 -> [_ _ _ w451 _]
          tunnel: w345 -> [_ _ _ _ _]
          tunnel: w344 -> [w445 _ _ _ _]
          tunnel: [w445 _ _ _ _] -> w343
          event Timeout {
            n111 = event-data() -> ()  [unwired: 1 in, 1 out]
          }
          event "Clear all charts": Value Change {
            (unwired) T33 [] ("History Data")
            w448 = cluster{dbl}[] [] ("History Data")
            w449 = cluster{"Resistance":sgl}[] [] ("History Data")
            w446 = dbl[] [] ("History Data")
            n112 = event-data() -> ()  [unwired: 1 in, 1 out]
            n113 = property on="K-6430" class="WFChart (strict)"("History Data"=w449) -> ()  [unwired: 2 in, 2 out]
            n114 = property on="arduino qcm 1" class="WFChart (strict)"("History Data"=w446) -> ()  [unwired: 2 in, 2 out]
            n115 = property on="Waveform Chart" class="WFChart (strict)"("History Data"=w448) -> ()  [unwired: 2 in, 2 out]
            n116 = property on="arduino qcm 6" class="WFChart (strict)"("History Data"=w446) -> ()  [unwired: 2 in, 2 out]
            n117 = property on="arduino qcm 3" class="WFChart (strict)"("History Data"=w446) -> ()  [unwired: 2 in, 2 out]
            n118 = property on="QCM plot" class="WFChart (strict)"("History Data"=cluster{dbl, "Resistance out":dbl}[] []) -> ()  [unwired: 2 in, 2 out]
            n119 = property on="K-2100 (Ohm)" class="WFChart (strict)"("History Data"=w449) -> ()  [unwired: 2 in, 2 out]
            n120 = property on="arduino qcm 4" class="WFChart (strict)"("History Data"=w446) -> ()  [unwired: 2 in, 2 out]
            n121 = property on="K-2420" class="WFChart (strict)"("History Data"=w449) -> ()  [unwired: 2 in, 2 out]
            n122 = property on="pressure chart" class="WFChart (strict)"("History Data"=w448) -> ()  [unwired: 2 in, 2 out]
            n123 = property on="arduino qcm 2" class="WFChart (strict)"("History Data"=w446) -> ()  [unwired: 2 in, 2 out]
            n124 = property on="arduino qcm 5" class="WFChart (strict)"("History Data"=w446) -> ()  [unwired: 2 in, 2 out]
          }
          event "Sequence cluster.Clear sequence": Value Change {
            n125 = event-data() -> ()  [unwired: 1 in, 1 out]
            n126 = property on="User-defined\nsequence" class="Tbl (strict)"("Value"=string[][] []) -> ()  [unwired: 2 in, 2 out]
          }
          event "Sequence cluster.Save sequence": Value Change {
            n127 = event-data() -> ()  [unwired: 1 in, 1 out]
            n128 = call-poly <vilib>:"Write To Spreadsheet File.vi"("2D data"=w451) -> ()  [unwired: 7 in, 1 out]
          }
          event "Sequence cluster.Import sequence file": Value Change {
            n129 = event-data() -> ()  [unwired: 1 in, 1 out]
            n130 = call-poly <vilib>:"Read From Spreadsheet File.vi"() -> ("all rows"=w452:string[][])  [unwired: 7 in, 4 out]
            n131 = property on="User-defined\nsequence" class="Tbl (strict)"("Value"=w452) -> ()  [unwired: 2 in, 2 out]
          }
        }
        n132 = Unbundle(w300) -> ("press/RH/gas/vapor"=w299:T34, "Cluster"=w298:T35)
        n133 = Divide(x=w390, y=T11 {"f"=1000000.0, "f"=1000000.0, "f"=1000000.0, "f"=1000000.0, "f"=1000000.0, "f 2"=1000000.0}) -> (x/y=w365:cluster{dbl, dbl, dbl, dbl, dbl, dbl})
        n134 = Unbundle(w298) -> ("Valve position (%)"=w296:dbl, "read pressure"=w290:dbl, "read vapor flow"=w295:dbl, "read gas flow"=w294:dbl)
        n135 = case shown="True" w277 {
          tunnel: w365 -> [_ w431]
          frame False {
          }
          frame True {
            n136 = Unbundle(w431) -> (w430:dbl, w429:dbl, w428:dbl, w427:dbl, w426:dbl, w424:dbl)
            n137 = Bundle(w430, w430, w429, w429, w428, w428, w427, w427, w426, w426, w424, w424) -> (→"ArduinoQCM\ncluster":T36)  [unwired: 1 in]
          }
        }
        n138 = Unbundle("Data logging settings") -> ("Save during sequence only"=w376:bool, "Save now"=w378:bool, "sec between data points"=w364:dbl, "Save sample names"=w318:T37, "Experiment Notes"=w317:string)  [unwired: 1 out]
        n139 = property on="Valve position (%)" class="DigNum (strict)"("Value"=w296) -> ()  [unwired: 2 in, 2 out]
        n140 = Subtract(x=w362, y=w343) -> (x-y=w361:dbl)
        n141 = property on="read pressure" class="DigNum (strict)"("Value"=w290) -> ()  [unwired: 2 in, 2 out]
        n142 = And(x=w297, y=w376) -> (x .and. y?=w375:bool)
        n143 = Bundle("read pressure"=w290) -> (w289:cluster{"read pressure":dbl})  [unwired: 1 in]
        n144 = Divide(x=w361, y=60.0) -> (x/y=w335:dbl)
        "Elapsed time (min)" <- w335
        n145 = call "data_headers_subVI.vi"("Experiment Notes"=w317, "Sample names"=w318) -> ("data headers"=w391:string[])  [unwired: 9 in]
        n146 = property on="read vapor flow" class="DigNum (strict)"("Value"=w295) -> ()  [unwired: 2 in, 2 out]
        n147 = Multiply(x=w364, y=u32 1000 ("x")) -> (x*y=w400:dbl)
        n148 = Or(x=w375, y=w378) -> (x .or. y?=w372:bool)
        "saving data?" <- w372
        n149 = Wait (ms)(milliseconds to wait=w400) -> ()  [unwired: 1 out]
        n150 = property on="read gas flow" class="DigNum (strict)"("Value"=w294) -> ()  [unwired: 2 in, 2 out]
        n151 = property on="pressure chart" class="WFChart (strict)"("Value"=w289) -> ()  [unwired: 2 in, 2 out]
        n152 = Get Date/Time In Seconds() -> (seconds since 1Jan1904=w422:timestamp)
        n153 = Number To Engineering String ("elapsed time (min)")(4:w335) -> (0:w340:string)  [unwired: 3 in]
        n154 = Unbundle(w312) -> ("current  step # in"=w286:i32, "sequence end time in"=w311:timestamp, "Boolean"=w310:bool)
        n155 = Format Date/Time String(time format string (%c)="%Y-%m-%d %H:%M:%S%2u", seconds (now)=w422) -> (date/time string=w397:string)  [unwired: 1 in]
        n156 = Unbundle(w348) -> ("String data out"=w339:string, w338:string, w337:string, w336:string)
        n157 = Unbundle(w396) -> ("String"=w341:string, "String"=w399:string, "String"=w398:string)
        n158 = Unbundle(w332) -> ("String"=w331:string, "String"=w330:string)
        n159 = Unbundle(w299) -> ("pressure"=w388:string, "RH"=w387:string, "gas flow"=w386:string, "vapor flow"=w385:string)
        n160 = Unbundle ("arduino 1-6")(w280) -> ("mean"=w284:string, "mean"=w395:string, "mean"=w394:string, "mean"=w393:string, "mean"=w392:string, "mean"=w282:string)
        n161 = Increment(x=w286) -> (x+1=w285:i32)
        n162 = Build Array(w397, w340, w339, w338, w337, w336, w341, w399, w398, w331, w330, w388, w387, w386, w385, w283, w284, w395, w394, w393, w392, w282) -> (w405:string[])
        n163 = property on="Current\nstep" class="DigNum (strict)"("Value"=w285) -> ()  [unwired: 2 in, 2 out]
        "State date/time" <- w334
      }
      n164 = Unbundle(w85) -> (w84:bool, "VISA resource name out"=w83:refnum<visa-resource-name>, "error out"=w82:errorcluster)
      n165 = Unbundle(w81) -> ("Boolean"=w80:bool, "VISA out"=w79:refnum<visa-resource-name>, "error out"=w78:errorcluster)
      n166 = call-poly <vilib>:"Write To Spreadsheet File.vi"("1D data"=w49, "file path (dialog if empty)"=w66) -> ("new file path (Not A Path if cancelled)"=w70:path)  [unwired: 6 in]
      n167 = Unbundle(w59) -> (w64:bool, "VISA resource name out"=w63:refnum<visa-resource-name>, "error out"=w62:errorcluster)
      n168 = Unbundle(w27) -> ("Boolean"=w26:bool, "DAQ IDs in"=w25:T38)
      n169 = call "arduino_close_subIV.vi"("arduino 1-6 addresses and errors out"=w51, "arduinos on?"=w50) -> ()  [unwired: 10 in]
      n170 = case shown="True" w42 {
        tunnel: w41 -> [_ w100]
        tunnel: w40 -> [w97 w99]
        tunnel: [w97 w98] -> w39
        frame False {
        }
        frame True {
          n171 = call "Close.vi"("VISA resource name"=w100, "error in (no error)"=w99) -> ("error out"=w98:errorcluster)  [unwired: 17 in]
        }
      }
      n172 = flat-sequence {
        tunnel: w5 -> [w96]
        tunnel: [w96] -> w4
        frame #0 {
          n173 = property on="saving data?" class="Bool (strict)"("Value"=FALSE ("saving data?")) -> ()  [unwired: 2 in, 2 out]
        }
      }
      n174 = Unbundle(w76) -> ("Boolean"=w75:bool, "VISA resource name out"=w74:refnum<visa-resource-name>, "error out"=w73:errorcluster)
      n175 = case shown="True" w26 {
        tunnel: w25 -> [_ w128]
        tunnel: [errorcluster {"status"=FALSE, "code"=0, "source"=""} ("error out") w115] -> w34
        frame False {
        }
        frame True {
          n176 = Unbundle(w128) -> ("task out"=w127:refnum<k21>, "error out"=w126:errorcluster, "task out"=w125:refnum<k21>, "error out"=w124:errorcluster, "task out"=w123:refnum<k21>, "error out"=w122:errorcluster, "VISA Refnum out"=w121:refnum<visa-resource-name>, "error out"=w120:errorcluster)
          n177 = disable-structure shown="Disabled" {
            disable-tunnel: [w137 _] -> w119
            disable-tunnel: w127 -> [w136 _]
            disable-tunnel: w126 -> [w135 _]
            frame Disabled {
              n178 = call <vilib>:"DAQmx Stop Task.vi"("task/channels in"=w136, "error in"=w135) -> ("task out"=w138:refnum<k21>, "error out"=w139:errorcluster)  [unwired: 12 in]
              n179 = call <vilib>:"DAQmx Clear Task.vi"("task in"=w138, "error in"=w139) -> ("error out"=w137:errorcluster)  [unwired: 13 in]
            }
            frame Enabled {
            }
          }
          n180 = call <vilib>:"DAQmx Stop Task.vi"("task/channels in"=w125, "error in"=w124) -> ("task out"=w132:refnum<k21>, "error out"=w131:errorcluster)  [unwired: 12 in]
          n181 = call <vilib>:"DAQmx Stop Task.vi"("task/channels in"=w123, "error in"=w122) -> ("task out"=w133:refnum<k21>, "error out"=w134:errorcluster)  [unwired: 12 in]
          n182 = VISA Clear(VISA resource name=w121, error in (no error)=w120) -> (VISA resource name out=w130:refnum<visa-resource-name>, error out=w129:errorcluster)
          n183 = VISA Close(VISA resource name=w130, error in (no error)=w129) -> (error out=w116:errorcluster)
          n184 = call <vilib>:"DAQmx Clear Task.vi"("task in"=w132, "error in"=w131) -> ("error out"=w118:errorcluster)  [unwired: 13 in]
          n185 = call <vilib>:"DAQmx Clear Task.vi"("task in"=w133, "error in"=w134) -> ("error out"=w117:errorcluster)  [unwired: 13 in]
          n186 = Merge Errors(w119, w118, w117, w116) -> (w115:errorcluster)
        }
      }
      n187 = case shown="True" w84 {
        tunnel: w83 -> [_ w250]
        tunnel: w82 -> [w247 w249]
        tunnel: [w247 w248] -> w86
        frame False {
        }
        frame True {
          n188 = call "Enable Output.vi"("error in (no error)"=w249, "Enable Output (T: Enable)"=FALSE, "VISA resource name"=w250) -> ("error out"=w251:errorcluster, "VISA resource name out"=w253:refnum<visa-resource-name>)  [unwired: 7 in]
          n189 = call "Close.vi"("error in (no error)"=w251, "VISA resource name"=w253) -> ("error out"=w248:errorcluster)  [unwired: 9 in]
        }
      }
      n190 = case shown="True" w64 {
        tunnel: w63 -> [_ w163]
        tunnel: w62 -> [w161 w162]
        tunnel: [w161 w164] -> w58
        frame False {
        }
        frame True {
          n191 = call "Enable Output.vi"("error in (no error)"=w162, "Enable Output (F:Off)"=FALSE ("Output (F:Off)"), "VISA resource name"=w163) -> ("error out"=w165:errorcluster, "VISA resource name out"=w166:refnum<visa-resource-name>)  [unwired: 7 out]
          n192 = call "Close.vi"("error in (no error)"=w165, "VISA resource name"=w166) -> ("error out"=w164:errorcluster)  [unwired: 9 out]
        }
      }
      n193 = case shown="True" w80 {
        tunnel: w78 -> [w233 w236]
        tunnel: [w233 w235] -> w87
        tunnel: w79 -> [_ w234]
        frame False {
        }
        frame True {
          n194 = call "srsQcm200Close.vi"("error in"=w236, "Visa in"=w234) -> ("error out"=w235:errorcluster)  [unwired: 3 in]
        }
      }
      n195 = call-poly <vilib>:"Write To Spreadsheet File.vi"("append to file? (new file:F)"=TRUE, "2D data"=w53, "file path (dialog if empty)"=w70) -> ()  [unwired: 5 in, 1 out]
      n196 = case shown="True" w75 {
        tunnel: w74 -> [_ w203]
        tunnel: w73 -> [w200 w202]
        tunnel: [w200 w201] -> w72
        frame False {
        }
        frame True {
          n197 = VISA Close(VISA resource name=w203, error in (no error)=w202) -> (error out=w201:errorcluster)
        }
      }
      n198 = Merge Errors(w58, w72, w86, w39, w87, w4) -> (w93:errorcluster)
      n199 = call <vilib>:"Simple Error Handler.vi"("error in (no error)"=w34) -> ()  [unwired: 4 in, 5 out]
      n200 = call <vilib>:"Simple Error Handler.vi"("error in (no error)"=w93) -> ()  [unwired: 4 in, 5 out]
    }
  }
